vi "Custom User Message.vi"(6 "Button text (\"OK\")":string="OK", 7 "MSG":string) -> (1 "Ok?":bool)   [LabVIEW 2021]
panel:
  in  "OK":bool
  in  "Title":string
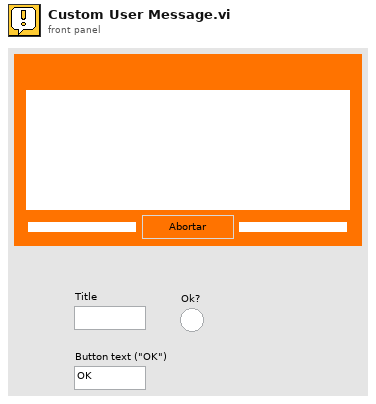
[diagram p1: front panel]
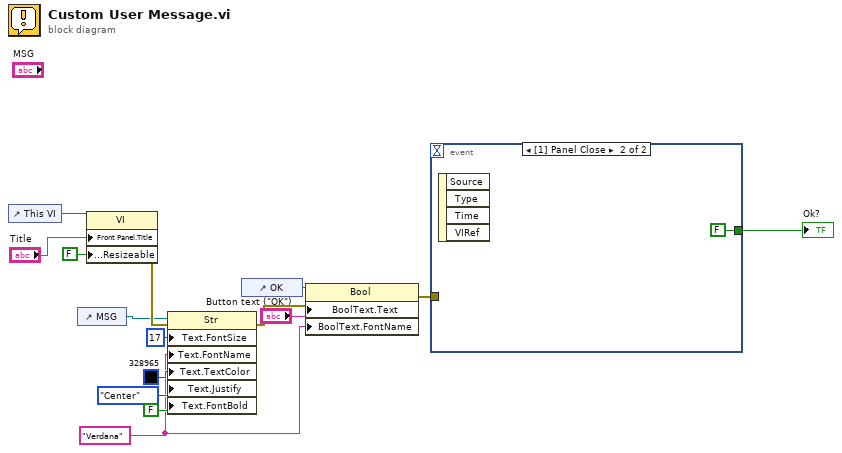
[diagram p0: block diagram]
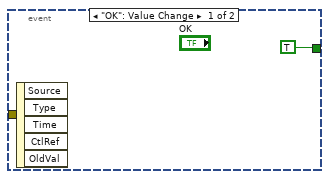
[diagram p2: hidden frame]
diagram:
  w1 = "Verdana" ("Text.Font:Name")
  n1 = control-ref of="This VI"() -> (w11:refnum<vi>)
  n2 = control-ref of="MSG"() -> (w2:refnum<vi>)
  n3 = property class="VI"(reference=w11, "Front Panel.Title"="Title", "Front Panel.Resizeable"=FALSE ("Front Panel Window:Resizable")) -> (error out=w9:errorcluster)  [unwired: 1 in, 1 out]
  n4 = property on="Property Node" class="Str"(reference=w2, error in=w9, "Text.FontSize"=u32 17 ("Text.Font:Size"), "Text.FontName"=w1, "Text.TextColor"=u32 328965 ("Text.Text Colors:Text Color"), "Text.Justify"=enum16{"Left", "Center", "Right"}."Center" ("Text.Justification"), "Text.FontBold"=FALSE ("Text.Font:Bold")) -> (error out=w4:errorcluster)  [unwired: 1 out]
  n5 = control-ref of="OK"() -> (w6:refnum<vi>)
  n6 = property on="Property Node" class="Bool"(reference=w6, error in=w4, "BoolText.Text"="Button text (\"OK\")", "BoolText.FontName"=w1) -> (error out=w3:errorcluster)  [unwired: 1 out]
  n7 = event shown="[1] Panel Close" {
    selector: _ -> [_ _]
    dyn-events: _ -> [_ _]
    timeout: _ -> [_ _]
    tunnel: [TRUE FALSE] -> w12
    tunnel: w3 -> [_ _]
    event "OK": Value Change {
      n8 = event-data() -> ()  [unwired: 6 out]
    }
    event Panel Close {
      n9 = event-data() -> ()  [unwired: 5 out]
    }
  }
  "Ok?" <- w12
